vi "Find Poles.vi"(0 "Particle Measurements":dbl[][](array[numeric])) -> (1 "Histogram Particle Xs":T3, 2 "Grouped Particles":T2, 3 "Grouped Partical Measurements":T1(array[cluster]), 4 "Spacing":dbl)   [LabVIEW 2013]
doc: "Use a histogram to group particles into up to three columns based on particle density."
uses:
  Gridded Particles.ctl
  <vilib>/Analysis/baseanly.llb/Mean (DBL).vi
  <vilib>/Analysis/NI_AALBase.lvlib
panel:
  out "Histogram of Xs":T3(graph)
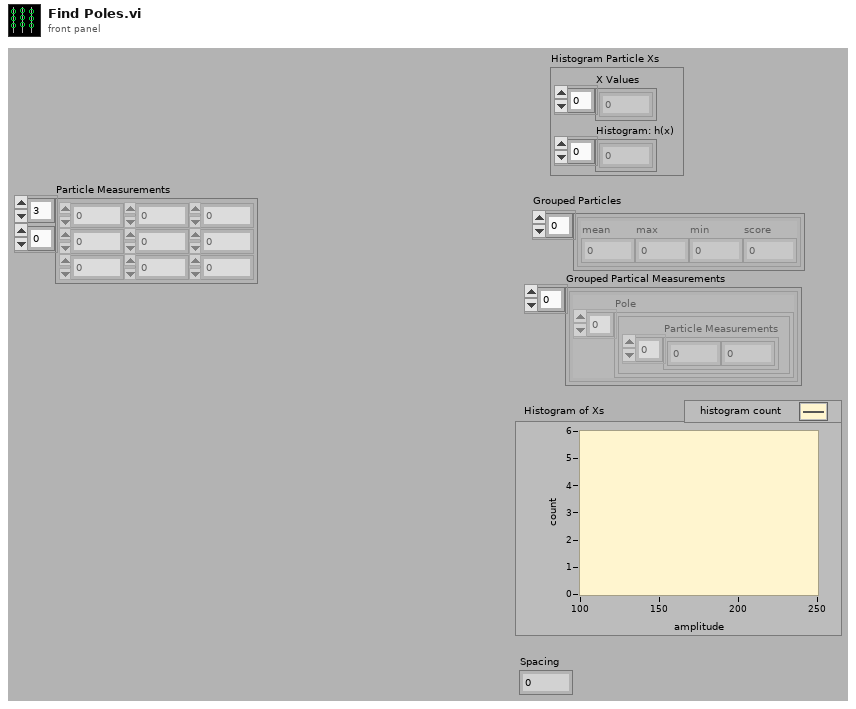
[diagram p1: front panel]
types:
  T1 = cluster{"Pole":cluster{"Particle Measurements":dbl[]}[]}[]
  T2 = typedef "Gridded Particles.ctl" = cluster{"mean":dbl, "max":dbl, "min":dbl, "score":dbl}[]
  T3 = cluster{"X Values":dbl[], "Histogram: h(x)":i32[]}
  T4 = cluster{cluster{"Particle Measurements":dbl[]}[]}
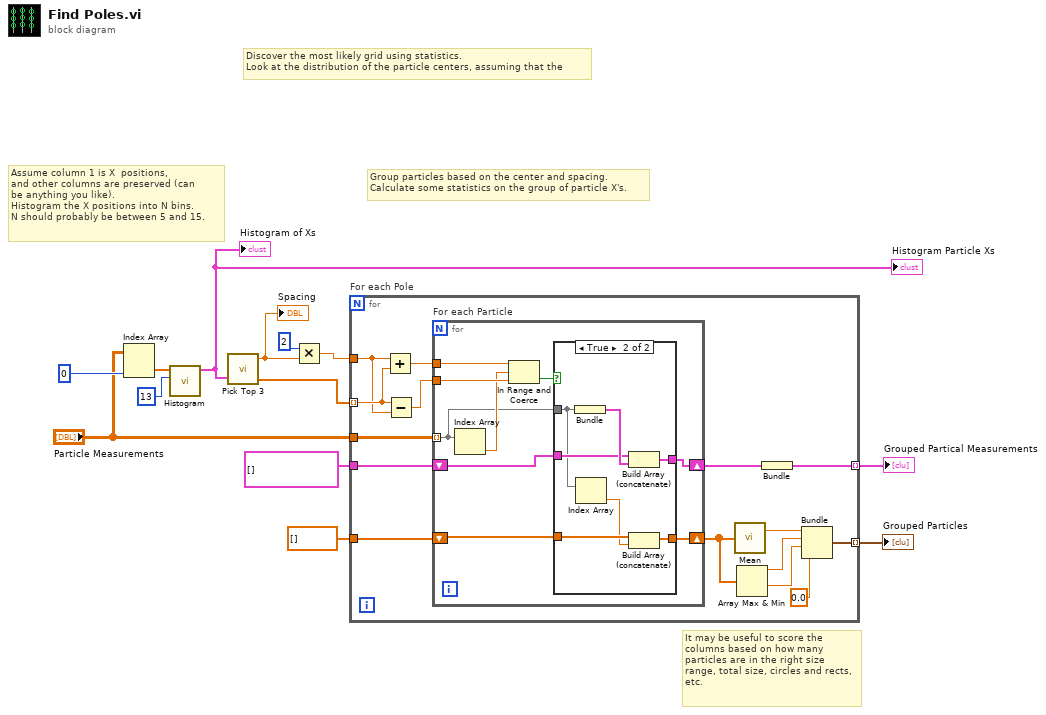
[diagram p0: block diagram]
diagram:
  # "It may be useful to score the\ncolumns based on how many\nparticles are in the right size\nrange, total size, circles and rects,\netc."
  # "Group particles based on the center and spacing.\nCalculate some statistics on the group of particle X's."
  # "Discover the most likely grid using statistics.\nLook at the distribution of the particle centers, assuming that the"
  # "Assume column 1 is X  positions,\nand other columns are preserved (can\nbe anything you like).\nHistogram the X positions into N bins.\nN should probably be between 5 and 15."
  n1 = Index Array(array="Particle Measurements", index (col)=0 ("disabled index (col)")) -> (element=w6:dbl[])  [unwired: 1 in]
  n2 = call <vilib>:"Histogram.vi"("intervals"=13, "X"=w6) -> ("Histogram Graph"=w11:T3)  [unwired: 9 out]
  "Histogram Particle Xs" <- w11
  "Histogram of Xs" <- w11
  n3 = call "Pick Top 3.vi"("Histogram Graph"=w11) -> ("spacing"=w1:dbl, "Top 3"=w9:dbl[])  [unwired: 1 in, 1 out]
  "Spacing" <- w1
  n4 = Multiply(x=2 ("Min Pts"), y=w1) -> (x*y=w4:dbl)
  n5 = for "For each Pole" {
    tunnel: w4 -> [w27]
    tunnel: w9 -> [w28] mode=indexing
    tunnel: "Particle Measurements" -> [w24]
    tunnel: cluster{"Particle Measurements":dbl[]}[] [] -> [w23]
    tunnel: dbl[] [] ("Particle Measurements") -> [w18]
    tunnel: [w16] -> w12 mode=indexing
    tunnel: [w14] -> w2 mode=indexing
    n6 = Add(x=w27, y=w28) -> (x+y=w26:dbl)
    n7 = Subtract(x=w28, y=w27) -> (x-y=w25:dbl)
    n8 = for "For each Particle" {
      tunnel: w26 -> [w37]
      tunnel: w25 -> [w36]
      tunnel: w24 -> [w33] mode=indexing
      shift-right: [w31] -> w15
      shift-left: w23 -> [w32]
      shift-right: [w29] -> w21
      shift-left: w18 -> [w30]
      n9 = Index Array(array=w33) -> (element=w35:dbl)  [unwired: 1 in]
      n10 = In Range and Coerce(upper limit=w37, x=w35, lower limit=w36) -> (In Range?=w34:bool)  [unwired: 1 out]
      n11 = case shown="True" w34 {
        tunnel: w33 -> [_ w43]
        tunnel: w32 -> [w39 w45]
        tunnel: [w39 w44] -> w31
        tunnel: w30 -> [w38 w42]
        tunnel: [w38 w41] -> w29
        frame False {
        }
        frame True {
          n12 = Bundle("Particle Measurements"=w43) -> (w46:cluster{"Particle Measurements":dbl[]})  [unwired: 1 in]
          n13 = Index Array(array=w43) -> (element=w40:dbl)  [unwired: 1 in]
          n14 = Build Array (concatenate)(w45, w46) -> (w44:cluster{"Particle Measurements":dbl[]}[])
          n15 = Build Array (concatenate)(w42, w40) -> (w41:dbl[])
        }
      }
    }
    n16 = call-poly <vilib>:"Mean.vi"("X"=w21) -> ("mean"=w22:dbl)  [unwired: 1 out]
    n17 = Array Max & Min(array=w21) -> (max value=w20:dbl, min value=w19:dbl)  [unwired: 2 out]
    n18 = Bundle(w15) -> (w14:T4)  [unwired: 1 in]
    n19 = Bundle("mean"=w22, w20, w19, "intervals"=0.0) -> (w16:cluster{"mean":dbl, dbl, dbl, "intervals":dbl})  [unwired: 1 out]
  }
  "Grouped Particles" <- w12
  "Grouped Partical Measurements" <- w2
